vi "section data extractor.vi"(2 "sections data":string[][](array[string])) -> (5 "#keys per section":i32[](array[numeric]), 6 "sections":string[](array[string]))   [LabVIEW 2024, in "Config Files Management.lvlib"]
uses:
  Config Files Management.lvlib
  section data row selector--ring.ctl
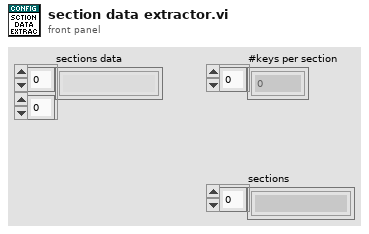
[diagram p1: front panel]
types:
  T1 = typedef "Config Files Management.lvlib/section data row selector--ring.ctl" = i32
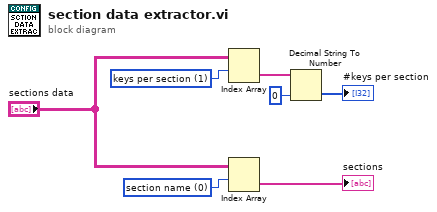
[diagram p0: block diagram]
diagram:
  w7 = T1 1 items=["section name", "keys per section"]
  w6 = T1 0 items=["section name", "keys per section"]
  n1 = Index Array(array="sections data", index (row)=w7) -> (element=w4:string[])  [unwired: 1 in]
  n2 = Index Array(array="sections data", index (row)=w6) -> (element=→"sections":string[])  [unwired: 1 in]
  n3 = Decimal String To Number(string=w4, default (0L)=0 ("default (0 I32)")) -> (number=→"#keys per section":i32[])  [unwired: 1 in, 1 out]
